vi "Byte_buffer_get_4.vi"(11 "queue out":refnum<queue>) -> (3 "Array":u8[](array[numeric]))   [LabVIEW 2017]
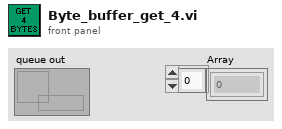
[diagram p1: front panel]
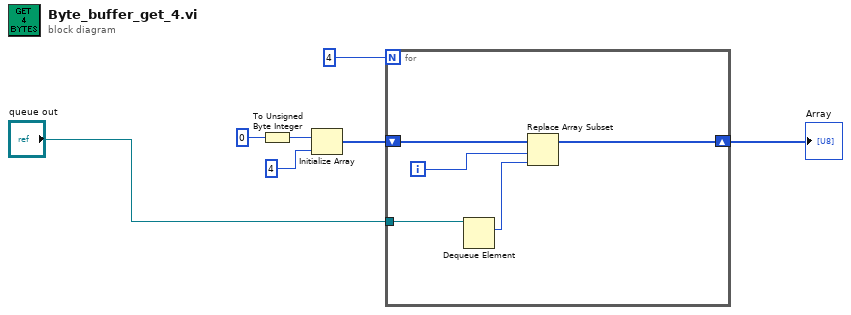
[diagram p0: block diagram]
diagram:
  n1 = To Unsigned Byte Integer(number=u8 0) -> (unsigned 8bit integer=w5:u8)
  n2 = Initialize Array(w5, 4 ("dimension size")) -> (w2:u8[])
  n3 = for {
    N: 4 -> [_]
    tunnel: "queue out" -> [w12]
    shift-right: [w8] -> w1
    shift-left: w2 -> [w9]
    i -> [w10]
    n4 = Dequeue Element(queue=w12) -> (element=w11:u8)  [unwired: 2 in, 3 out]
    n5 = Replace Array Subset(array=w9, new element=w11, index=w10) -> (w8:u8[])
  }
  "Array" <- w1
